vi "TransparencyEffect.vi"(7 "Operation":T1=enum."Hide 80%", 8 "error in":errorcluster, 11 "VI Ref in":refnum<vi>) -> (0 "error out":errorcluster)   [LabVIEW 2011]
uses:
  Controls/TransparencyEffectOperations.ctl
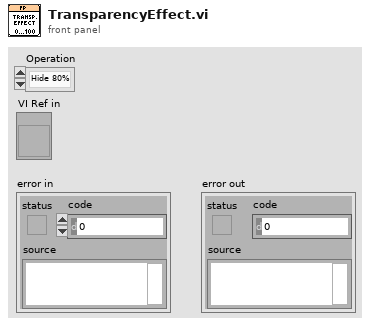
[diagram p1: front panel]
types:
  T1 = typedef "TransparencyEffectOperations.ctl" = enum16{"Show", "Hide 80%", "Hide All"}
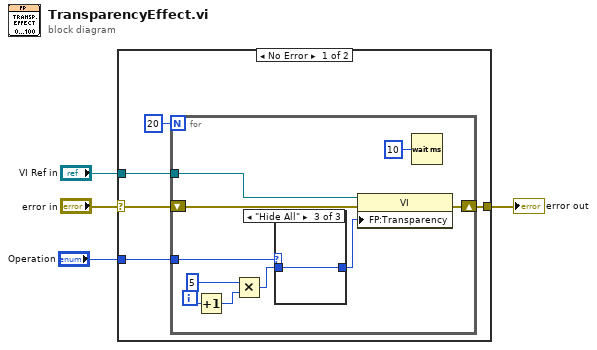
[diagram p0: block diagram]
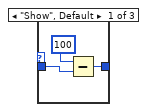
[diagram p2: hidden frame]
diagram:
  n1 = case shown="No Error" "error in" {
    selector: "error in" -> [w6 w25]
    tunnel: [w9 w25] -> w4
    tunnel: "VI Ref in" -> [w8 _]
    tunnel: "Operation" -> [w5 _]
    frame No Error {
      n2 = for {
        N: 20 -> [_]
        tunnel: w8 -> [w17]
        shift-right: [w16] -> w9
        shift-left: w6 -> [w15]
        tunnel: w5 -> [w10]
        i -> [w19]
        n3 = Increment(x=w19) -> (x+1=w14:i32)
        n4 = Multiply(x=5, y=w14) -> (x*y=w13:i32)
        n5 = case shown="\"Hide All\"" w10 {
          tunnel: w13 -> [w21 w23 w24]
          tunnel: [w20 w23 w24] -> w12
          frame "Show", Default {
            n6 = Subtract(x=100, y=w21) -> (x-y=w20:i32)
          }
          frame "Hide 80%" {
          }
          frame "Hide All" {
          }
        }
        n7 = property class="VI"(reference=w17, error in=w15, "FP:Transparency"=w12) -> (error out=w16:errorcluster)  [unwired: 1 out]
        n8 = Wait (ms)(milliseconds to wait=u32 10) -> ()  [unwired: 1 out]
      }
    }
    frame Error {
    }
  }
  "error out" <- w4
